vi "Cylinder coordinate sorter.vi"() -> ()   [LabVIEW 2015]
panel:
  out "Sensor no. cylinder":sgl[](array[numeric])=[0.0, 1.0, 2.0, 3.0, 4.0, 5.0, 6.0, 7.0, 8.0, 9.0, 10.0, 11.0, 12.0, 13.0, 14.0, 15.0, 16.0, 17.0, 18.0, 19.0]
  out "Tube no. cylinder":sgl[](array[numeric])=[1.0, 2.0, 3.0, 4.0, 5.0, 6.0, 7.0, 8.0, 9.0, 10.0, 11.0, 12.0, 13.0, 14.0, 15.0, 16.0, 17.0, 18.0, 19.0, 20.0]
  out "Winding no. cylinder":sgl[](array[numeric])=[1.0, 2.0, 3.0, 4.0, 5.0, 6.0, 7.0, 8.0, 9.0, 10.0, 11.0, 12.0, 13.0, 14.0, 15.0, 16.0, 17.0, 18.0, 19.0, 20.0]
  out "y/c cylinder":sgl[](array[numeric])=[0.25881904, 0.5, 0.70710677, 0.8660254, 0.9659258, 0.9659258, 0.8660254, 0.70710677, 0.5, 0.25881904, -0.25881904, -0.5, -0.70710677, -0.8660254, -0.9659258, -0.9659258, -0.8660254, -0.70710677, -0.5, -0.25881904]
  out "x/c cylinder":sgl[](array[numeric])=[0.9659258, 0.8660254, 0.70710677, 0.5, 0.25881904, -0.25881904, -0.5, -0.70710677, -0.8660254, -0.9659258, -0.9659258, -0.8660254, -0.70710677, -0.5, -0.25881904, 0.25881904, 0.5, 0.70710677, 0.8660254, 0.9659258]
  out "Cylinder: Winding sorted array":sgl[][](array[numeric])=[[0.0, 1.0, 1.0, 0.9659258, 0.25881904], [1.0, 2.0, 2.0, 0.8660254, 0.5], [2.0, 3.0, 3.0, 0.70710677, 0.70710677], [3.0, 4.0, 4.0, 0.5, 0.8660254], [4.0, 5.0, 5.0, 0.25881904, 0.9659258], [5.0, 6.0, 6.0, -0.25881904, 0.9659258], [6.0, 7.0, 7.0, -0.5, 0.8660254], [7.0, 8.0, 8.0, -0.70710677, 0.70710677], [8.0, 9.0, 9.0, -0.8660254, 0.5], [9.0, 10.0, 10.0, -0.9659258, 0.25881904], [10.0, 11.0, 11.0, -0.9659258, -0.25881904], [11.0, 12.0, 12.0, -0.8660254, -0.5], [12.0, 13.0, 13.0, -0.70710677, -0.70710677], [13.0, 14.0, 14.0, -0.5, -0.8660254], [14.0, 15.0, 15.0, -0.25881904, -0.9659258], [15.0, 16.0, 16.0, 0.25881904, -0.9659258], [16.0, 17.0, 17.0, 0.5, -0.8660254], [17.0, 18.0, 18.0, 0.70710677, -0.70710677], [18.0, 19.0, 19.0, 0.8660254, -0.5], [19.0, 20.0, 20.0, 0.9659258, -0.25881904]]
  in  "Cylinder: Sensor no.; Tube no.; Winding no.; x/c; y/c":string="0\t1\t1\t0.965925826\t0.258819045\n1\t2\t2\t0.866025404\t0.5\n2\t3\t3\t0.707106781\t0.707106781\n3\t4\t4\t0.5\t0.866025404\n4\t5\t5\t0.258819045\t0.965925826\n5\t6\t6\t-0.258819045\t0.965925826\n6\t7\t7\t-0.5\t0.866025404\n7\t8\t8\t-0.707106781\t0.707106781\n8\t9\t9\t-0.866025404\t0.5\n9\t10\t10\t-0.965925826\t0.258819045\n10\t11\t11\t-0.965925826\t-0.258819045\n11\t12\t12\t-0.866025404\t-0.5\n12\t13\t13\t-0.707106781\t-0.707106781\n13\t14\t14\t-0.5\t-0.866025404\n14\t15\t15\t-0.258819045\t-0.965925826\n15\t16\t16\t0.258819045\t-0.965925826\n16\t17\t17\t0.5\t-0.866025404\n17\t18\t18\t0.707106781\t-0.707106781\n18\t19\t19\t0.866025404\t-0.5\n19\t20\t20\t0.965925826\t-0.258819045\n"
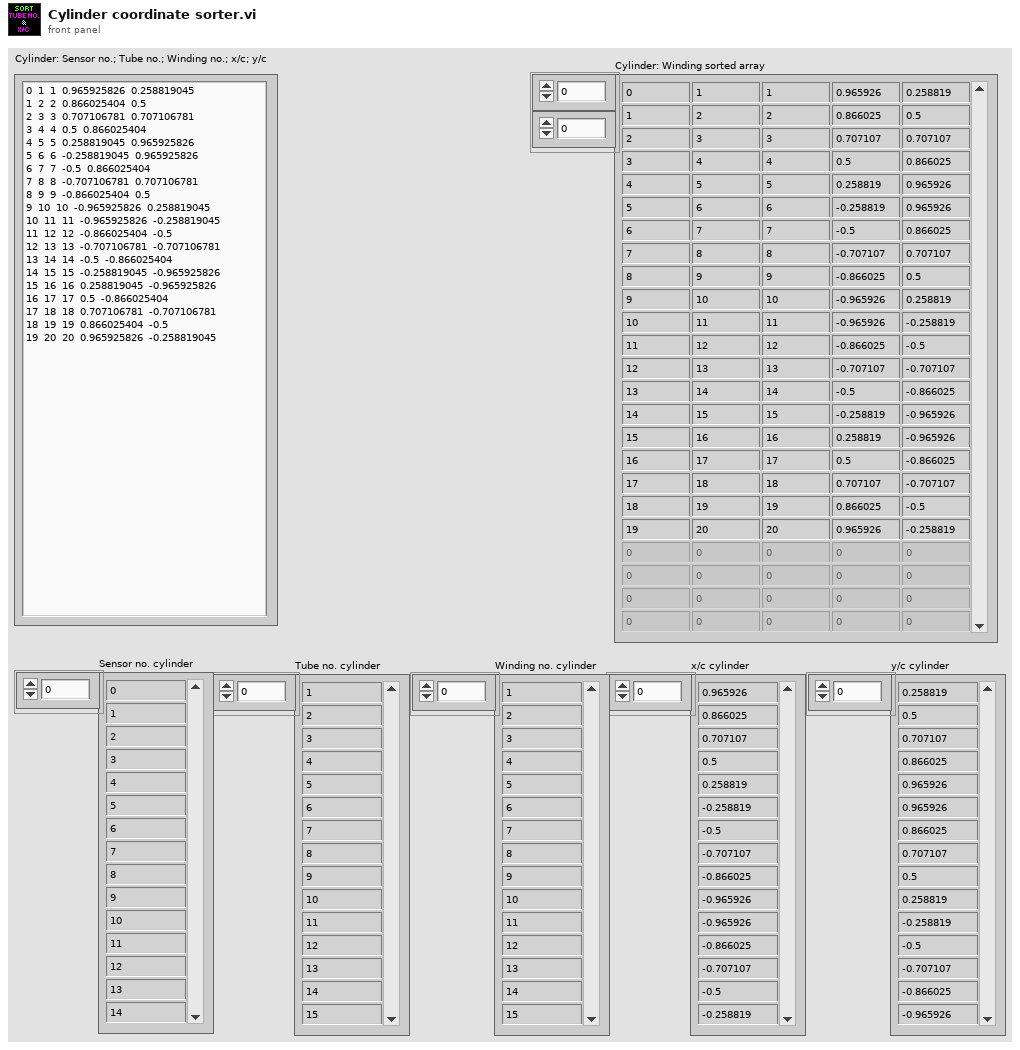
[diagram p1: front panel]
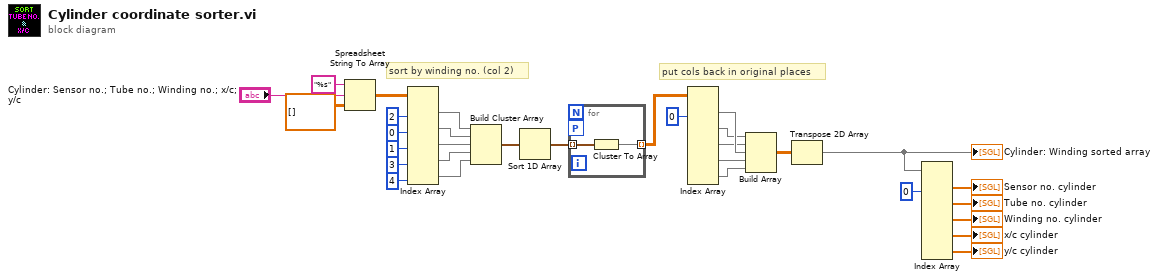
[diagram p0: block diagram]
diagram:
  # "sort by winding no. (col 2)"
  # "put cols back in original places"
  n1 = Spreadsheet String To Array(format string="%s", spreadsheet string="Cylinder: Sensor no.; Tube no.; Winding no.; x/c; y/c", array type (2D Dbl)=sgl[][] []) -> (array=w29:sgl[][])  [unwired: 1 in]
  n2 = Index Array(array=w29, index (col) #1=2 ("disabled index (col)"), index (col) #2=0 ("index (col)"), index (col) #3=1 ("index (col)"), index (col) #4=3 ("index (col)"), index (col) #5=4 ("index (col)")) -> (element #1=w27:sgl[], element #2=w26:sgl[], element #3=w21:sgl[], element #4=w20:sgl[], element #5=w19:sgl[])  [unwired: 5 in]
  n3 = Build Cluster Array(w27, w26, w21, w20, w19) -> (w25:cluster{sgl, sgl, sgl, sgl, sgl}[])
  n4 = Sort 1D Array(array=w25) -> (sorted array=w24:cluster{sgl, sgl, sgl, sgl, sgl}[])
  n5 = for {
    tunnel: w24 -> [w33] mode=indexing
    tunnel: [w32] -> w13 mode=indexing
    workers-P: _ -> [_]
    n6 = Cluster To Array(cluster=w33) -> (array=w32:sgl[])
  }
  n7 = Index Array(array=w13, index (col) #1=0 ("disabled index (col)")) -> (element #1=w12:sgl[], element #2=w11:sgl[], element #3=w10:sgl[], element #4=w9:sgl[], element #5=w8:sgl[])  [unwired: 9 in]
  n8 = Build Array(w11, w10, w12, w9, w8) -> (w7:sgl[][])
  n9 = Transpose 2D Array(2D array=w7) -> (transposed array=w6:sgl[][])
  "Cylinder: Winding sorted array" <- w6
  n10 = Index Array(array=w6, index (col) #1=0 ("disabled index (col)")) -> (element #1=→"Sensor no. cylinder":sgl[], element #2=→"Tube no. cylinder":sgl[], element #3=→"Winding no. cylinder":sgl[], element #4=→"x/c cylinder":sgl[], element #5=→"y/c cylinder":sgl[])  [unwired: 9 in]
